vi "System Identification.vi"() -> ()   [LabVIEW 2015]
uses:
  <vilib>/FPGAPlugInAG/myRIO-1900/niLvFpga_Open_myRIO-1900.vi
  <vilib>/rvi/interface/common/dynamic/niFpgaDynamicAddResources.vi
  <vilib>/Utility/error.llb/Error Cluster From Error Code.vi
  <vilib>/rvi/errors/niLvFpgaAdjustHostInterfaceError.vi
  <vilib>/Utility/file.llb/Write Delimited Spreadsheet (I64).vi
  <vilib>/Utility/file.llb/Write Delimited Spreadsheet (DBL).vi
  <vilib>/FPGAPlugInAG/Dynamic/niLvFpga_Close_Dynamic.vi
  <vilib>/rvi/interface/nirviOpenFPGA/nirviOpenFPGA.xnode
  FPGA Bitfiles/ACC20115_FPGATarget_CurrentControlle_Dt5vFgOzYtY.lvbitx
  Current Controller.vi
  <vilib>/rvi/interface/nirviReadWriteControl/nirviReadWriteControl.xnode
  <vilib>/rvi/interface/nirviCloseFPGA/nirviCloseFPGA.xnode
  <vilib>/rvi/interface/Simulation/niFpgaSimulationCallBeginRW.vi
  NiFpgaLv.dll
panel:
  out "Current (mA)":i32(graph)
  out "Received Data":dbl(graph)
  out "Status?":bool
  out "error out":errorcluster
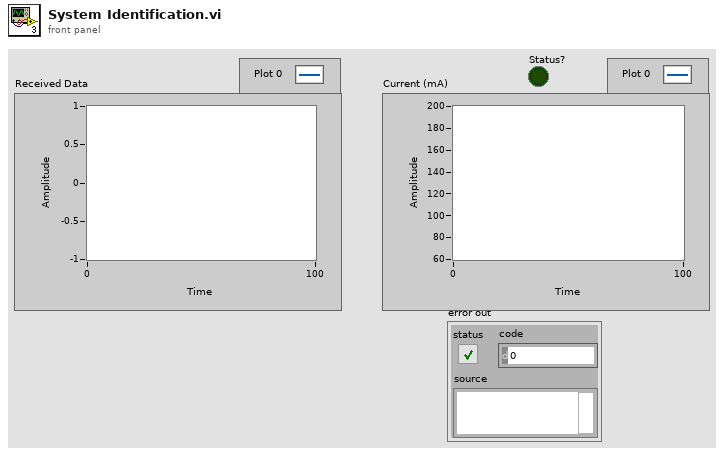
[diagram p1: front panel]
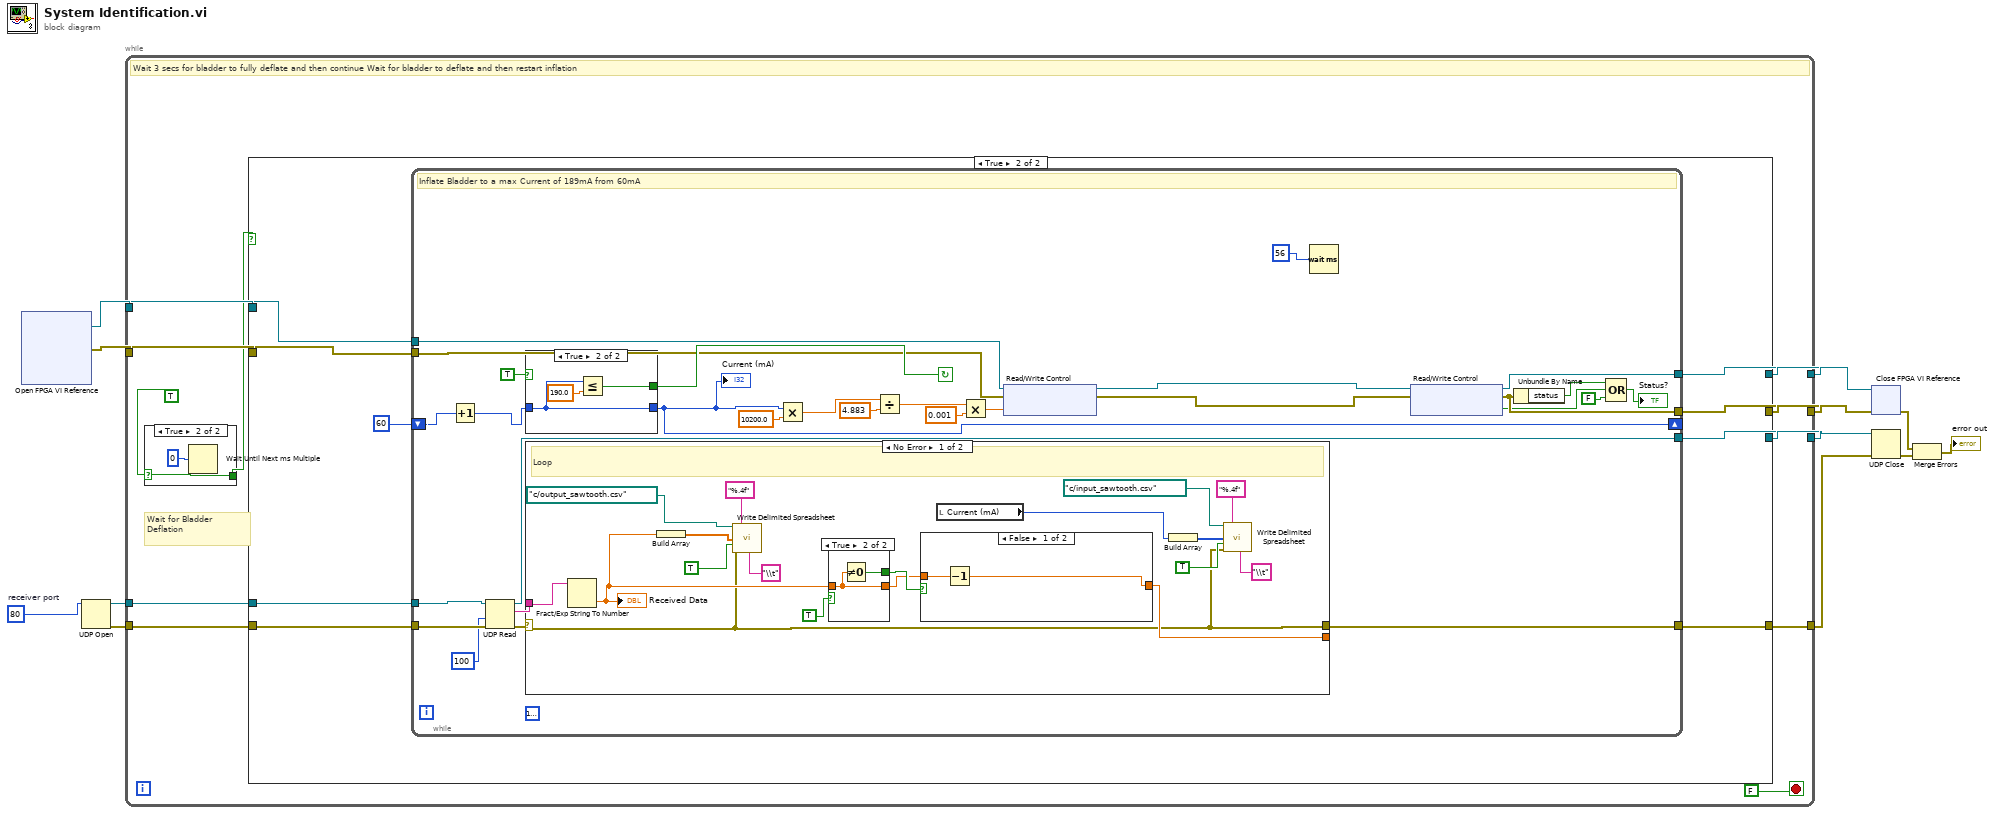
[diagram p0: block diagram]
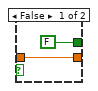
[diagram p5: hidden frame]
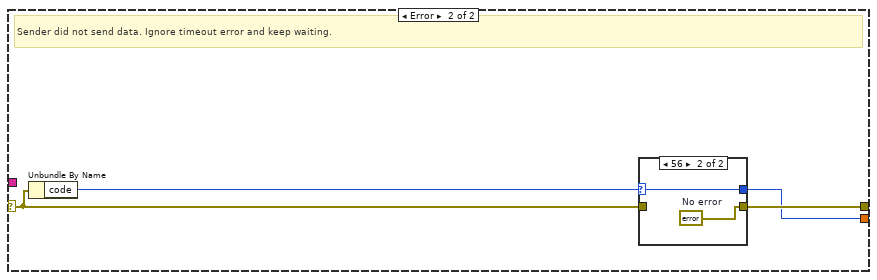
[diagram p6: hidden frame]
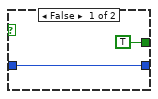
[diagram p8: hidden frame]
diagram:
  w12 = u16 80  # receiver port
  n1 = xnode "Open FPGA VI Reference"() -> ("FPGA VI Reference Out"=w2:refnum<k20>, "error out"=w5:errorcluster)  [unwired: 2 in]
  n2 = UDP Open(11:w12) -> (port=w11:refnum<k16>, 0:w10:errorcluster)  [unwired: 4 in, 1 out]
  n3 = while {
    tunnel: w2 -> [w17]
    tunnel: [w18] -> w3
    tunnel: w5 -> [w20]
    tunnel: [w19] -> w4
    tunnel: w11 -> [w23]
    tunnel: [w21] -> w9
    tunnel: w10 -> [w22]
    tunnel: [w14] -> w1
    stop <- FALSE stop-if-true
    # "Wait for Bladder Deflation"
    # "Wait 3 secs for bladder to fully deflate and then continue Wait for bladder to deflate and then restart inflation"
    n4 = case shown="True" TRUE {
      selector: TRUE -> [w24 w25]
      tunnel: [w24 w25] -> w15
      frame False {
      }
      frame True {
        n5 = Wait Until Next ms Multiple(millisecond multiple=u32 0) -> ()  [unwired: 1 out]
      }
    }
    n6 = case shown="True" w15 {
      tunnel: w23 -> [w28 w39]
      tunnel: w22 -> [w27 w38]
      tunnel: [w28 w37] -> w21
      tunnel: w20 -> [w29 w36]
      tunnel: [w29 w35] -> w19
      tunnel: [w30 w34] -> w18
      tunnel: w17 -> [w30 w33]
      tunnel: [w27 w31] -> w14
      frame False {
      }
      frame True {
        n7 = while {
          tunnel: w39 -> [w68]
          tunnel: [w66] -> w37
          tunnel: w38 -> [w67]
          tunnel: w33 -> [w62]
          tunnel: [w63] -> w34
          tunnel: w36 -> [w40]
          tunnel: [w64] -> w35
          shift-right: [w41] -> _
          shift-left: 60 -> [w44]
          tunnel: [w46] -> w31
          stop <- w49 continue-if-true
          (unwired) u32 16777216
          # "Inflate Bladder to a max Current of 189mA from 60mA"
          n8 = Increment(x=w44) -> (x+1=w43:i32)
          n9 = UDP Read(connection ID=w68, timeout ms (25000)=100, 8:w67) -> (data out=w48:string, error out=w47:errorcluster, 3:w66:refnum<k16>)  [unwired: 3 out]
          n10 = case shown="True" TRUE {
            tunnel: w43 -> [w103 w104]
            tunnel: [TRUE w105] -> w49
            tunnel: [w103 w104] -> w41
            frame False {
            }
            frame True {
              n11 = Less Or Equal?(x=w104, y=190.0) -> (x <= y?=w105:bool)
            }
          }
          "Current (mA)" <- w41
          n12 = case shown="No Error" w47 {
            selector: w47 -> [w69 w96]
            tunnel: w48 -> [w82 _]
            tunnel: [w69 w95] -> w46
            tunnel: [w83 w94] -> _
            frame No Error {
              # "Loop"
              n13 = Fract/Exp String To Number(string=w82) -> (number=w77:dbl)  [unwired: 3 in, 1 out]
              "Received Data" <- w77
              n14 = Build Array(w77) -> (w76:dbl[])
              n15 = call-poly <vilib>:"Write Delimited Spreadsheet.vi"("file path (dialog if empty)"=path "c:/output_sawtooth.csv", "format (%.3f)"="%.4f" ("format (%d)"), "1D data"=w76, "append to file? (F)"=TRUE ("append to file? (new file:F)"), "error in (no error)"=w69, "delimiter (\\t)"="\\t" ("delimiter (\\t)")) -> ()  [unwired: 8 in, 2 out]
              n16 = case shown="True" TRUE {
                tunnel: w77 -> [w90 w92]
                tunnel: [FALSE w93] -> w85
                tunnel: [w90 w92] -> w84
                frame False {
                }
                frame True {
                  n17 = Not Equal To 0?(x=w92) -> (x != 0?=w93:bool)
                }
              }
              n18 = case shown="False" w85 {
                tunnel: w84 -> [w88 w89]
                tunnel: [w87 w89] -> w83
                frame False {
                  n19 = Decrement(x=w88) -> (x-1=w87:dbl)
                }
                frame True {
                }
              }
              n20 = local read "Current (mA)"() -> (w71:i32)
              n21 = Build Array(w71) -> (w70:i32[])
              n22 = call-poly <vilib>:"Write Delimited Spreadsheet.vi"("file path (dialog if empty)"=path "c:/input_sawtooth.csv", "format (%d)"="%.4f", "1D data"=w70, "append to file? (F)"=TRUE ("append to file? (new file:F)"), "error in (no error)"=w69, "delimiter (\\t)"="\\t" ("delimiter (\\t)")) -> ()  [unwired: 8 in, 2 out]
            }
            frame Error {
              # "Sender did not send data. Ignore timeout error and keep waiting."
              n23 = Unbundle By Name(w96) -> ("code"=w97:i32)
              n24 = case shown="56" w97 {
                selector: w97 -> [w98 w100]
                tunnel: w96 -> [w99 _]
                tunnel: [w99 w101] -> w95
                tunnel: [w98 w100] -> w94
                frame Default {
                }
                frame 56 {
                  w101 = errorcluster {"status"=FALSE, "code"=0, "source"=""}  # No error
                }
              }
            }
          }
          n25 = Multiply(x=w41, y=10200.0) -> (x*y=w51:dbl)
          n26 = Divide(x=w51, y=4.883) -> (x/y=w54:dbl)
          n27 = Multiply(x=w54, y=0.001) -> (x*y=w42:dbl)
          n28 = xnode "Read/Write Control"("FPGA VI Reference In"=w62, "error in"=w40, "DAC Inlet Valve"=w42) -> ("FPGA VI Reference Out"=w61:refnum<k20>, "error out"=w60:errorcluster)
          n29 = Wait (ms)(milliseconds to wait=i64 56 ("Period")) -> ()  [unwired: 1 out]
          n30 = xnode "Read/Write Control"("FPGA VI Reference In"=w61, "error in"=w60) -> ("FPGA VI Reference Out"=w63:refnum<k20>, "error out"=w64:errorcluster, "Inlet Overflow?"=w59:bool)
          n31 = Unbundle By Name(w64) -> ("status"=w57:bool)
          n32 = Compound Arithmetic op=OR(w57, w59, FALSE ("value")) -> (→"Status?":bool)
        }
      }
    }
  }
  n33 = xnode "Close FPGA VI Reference"("FPGA VI Reference In"=w3, "error in"=w4) -> ("error out"=w6:errorcluster)
  n34 = UDP Close(connection ID=w9, 8:w1) -> (error out=w8:errorcluster)  [unwired: 1 out]
  n35 = Merge Errors(w6, w8) -> (→"error out":errorcluster)
